vi "Facade.vi"(0 "Data In":T4 caption="数据输入", 2 "Display State In":T2 caption="显示状态输入", 3 "Container State":T3 caption="容器状态") -> (6 "Data Out":T4 caption="数据输出", 7 "Display State Out":T2 caption="显示状态输出", 8 "Action":T1 caption="动作")   [LabVIEW 2016, in "PairTable.xctl"]
uses:
  PairTable.xctl
  Data.ctl
  <vilib>/_xctls/Container State.ctl
  Status.ctl
  <vilib>/_xctls/Action.ctl
  <vilib>/_xctls/XControlSupport.lvlib
panel:
  in  "?":i32(listbox)
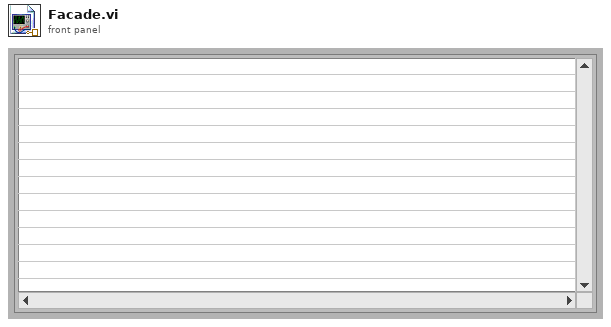
[diagram p1: front panel]
types:
  T1 = typedef "XControlSupport.lvlib/Action.ctl" = cluster{"Data Changed?":bool, "State Changed?":bool, "Action Name":string}
  T2 = typedef "PairTable.xctl/Status.ctl" = cluster{"Numeric":dbl}
  T3 = typedef "XControlSupport.lvlib/Container State.ctl" = cluster{"Indicator?":bool, "Run Mode?":bool, " Refnum":refnum<vi>}
  T4 = typedef "PairTable.xctl/Data.ctl" = cluster{"c":string, "l":string}[]
  T5 = typedef "LVBoundsTypeDef.ctl" = cluster{"Width":u32, "Height":u32}
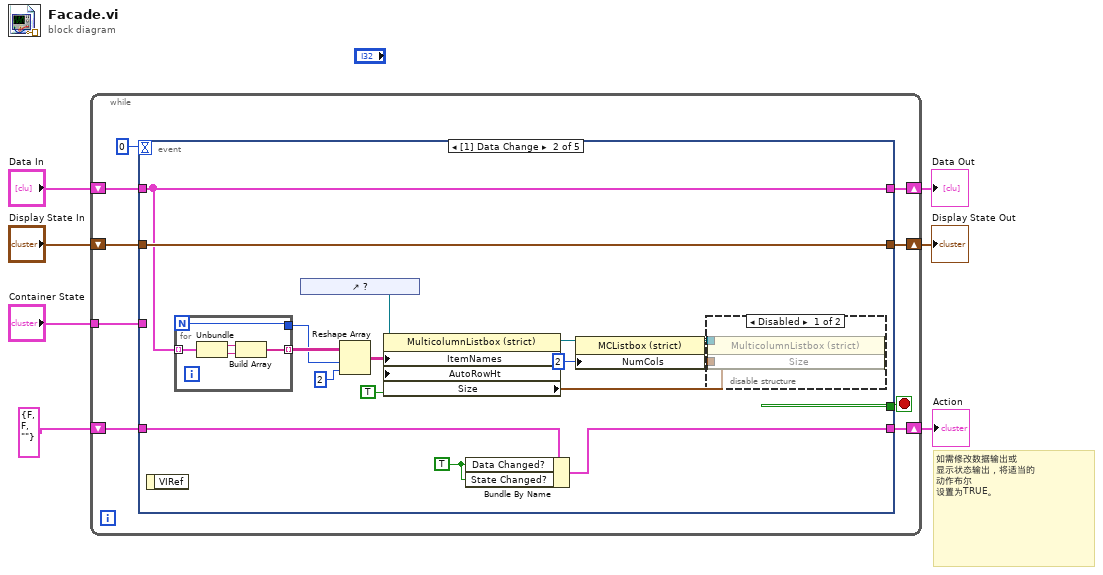
[diagram p0: block diagram]
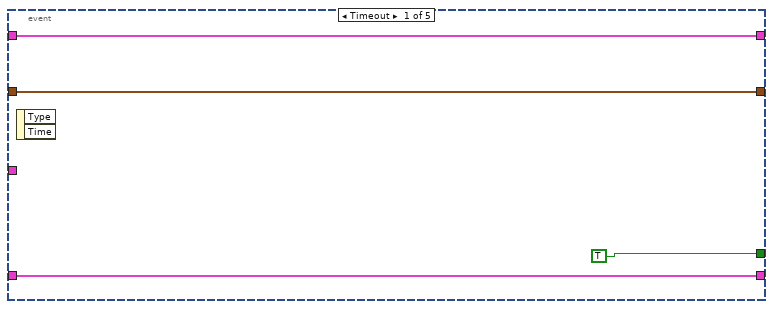
[diagram p2: hidden frame]
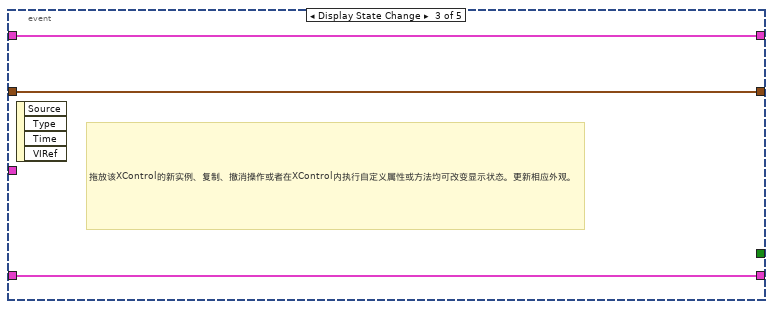
[diagram p4: hidden frame]
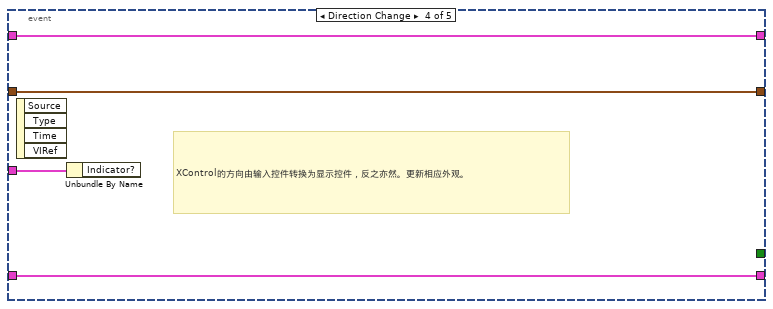
[diagram p5: hidden frame]
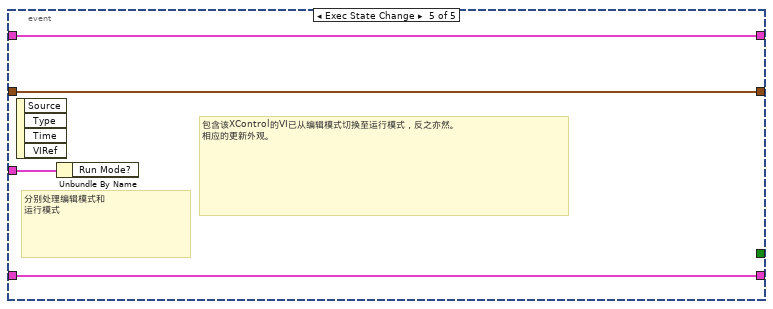
[diagram p6: hidden frame]
diagram:
  # "如需修改数据输出或\n显示状态输出，将适当的\n动作布尔\n设置为TRUE。"
  n1 = while {
    shift-right: [w15] -> w4
    shift-left: "Display State In" -> [w16]
    tunnel: "Container State" -> [w12]
    shift-right: [w10] -> w7
    shift-left: "Data In" -> [w11]
    shift-right: [w8] -> w2
    shift-left: T1 {"Data Changed?"=FALSE, "State Changed?"=FALSE, "Action Name"=""} ("Action") -> [w9]
    stop <- w14 stop-if-true
    n2 = event shown="[1] Data Change" {
      selector: _ -> [_ _ _ _ _]
      dyn-events: _ -> [_ _ _ _ _]
      timeout: 0 -> [_ _ _ _ _]
      tunnel: w16 -> [w18 w35 w45 w48 w52]
      tunnel: [w18 w35 w45 w48 w52] -> w15
      tunnel: [TRUE _ _ _ _] -> w14
      tunnel: w12 -> [_ _ _ w49 w53]
      tunnel: w11 -> [w17 w29 w44 w47 w51]
      tunnel: [w17 w29 w44 w47 w51] -> w10
      tunnel: [w19 w26 w43 w46 w50] -> w8
      tunnel: w9 -> [w19 w27 w43 w46 w50]
      event Timeout {
        n3 = event-data() -> ()  [unwired: 3 out]
      }
      event Data Change {
        w25 = TRUE ("Data Changed?")
        n4 = event-data() -> ()  [unwired: 2 out]
        n5 = for {
          N -> [w38]
          tunnel: w29 -> [w42] mode=indexing
          tunnel: [w39] -> w34 mode=indexing
          tunnel: [w38] -> w30
          n6 = Unbundle(w42) -> ("c"=w41:string, "l"=w40:string)
          n7 = Build Array(w41, w40) -> (w39:string[])
        }
        n8 = control-ref of="?"() -> (w28:refnum<vi>)
        n9 = Reshape Array(w34, w30, 2 ("维数大小")) -> (w32:string[][])
        n10 = property class="MulticolumnListbox (strict)"(reference=w28, "ItemNames"=w32, "AutoRowHt"=TRUE ("允许编辑单元格")) -> (reference out=w31:refnum<vi>, "Size"=w21:T5)  [unwired: 1 in, 1 out]
        n11 = Bundle By Name(cluster=w27, "Data Changed?"=w25, "State Changed?"=w25) -> (w26:T1)
        n12 = property class="MCListbox (strict)"(reference=w31, "NumCols"=u32 2 ("列数")) -> (reference out=w23:refnum<vi>)  [unwired: 1 in, 1 out]
        n13 = disable-structure shown="Disabled" {
          disable-tunnel: w23 -> [w37 _]
          disable-tunnel: w21 -> [w36 _]
          frame Disabled {
            n14 = property class="MulticolumnListbox (strict)"(reference=w37, "Size"=w36) -> ()  [unwired: 1 in, 2 out]
          }
          frame Enabled {
          }
        }
      }
      event Display State Change {
        # "拖放该XControl的新实例、复制、撤消操作或者在XControl内执行自定义属性或方法均可改变显示状态。更新相应外观。"
        n15 = event-data() -> ()  [unwired: 5 out]
      }
      event Direction Change {
        # "XControl的方向由输入控件转换为显示控件，反之亦然。更新相应外观。"
        n16 = event-data() -> ()  [unwired: 5 out]
        n17 = Unbundle By Name(w49) -> ()  [unwired: 1 out]
      }
      event Exec State Change {
        # "包含该XControl的VI已从编辑模式切换至运行模式，反之亦然。\n相应的更新外观。"
        # "分别处理编辑模式和\n运行模式"
        n18 = event-data() -> ()  [unwired: 5 out]
        n19 = Unbundle By Name(w53) -> ()  [unwired: 1 out]
      }
    }
  }
  "Display State Out" <- w4
  "Data Out" <- w7
  "Action" <- w2
